vi "rtAppMain.vi"() -> ()   [LabVIEW 2012]
doc: "Top-level application."
uses:
  Typedefs/ContextID.ctl
  ContextIDFactory/ContextIDFactory.lvclass
  ContextThisComponent/ContextThisComponent.lvclass
  InvokerThisComponent/InvokerThisComponent.lvclass
  CommandFactory/CommandFactory.lvclass
  StateFactory/StateFactory.lvclass
  Model/Model/Model.lvclass
  C/Program Files (x86)/National Instruments/LabVIEW 2012/user.lib/Common/ComponentModel/ComponentModel/UserEventBasedController/UserEventBasedController.lvclass
  C/Program Files (x86)/National Instruments/LabVIEW 2012/user.lib/Common/ComponentModel/ComponentModelRT/IRQHandler/IRQHandler/IRQHandler.lvclass
  C/Program Files (x86)/National Instruments/LabVIEW 2012/user.lib/Common/ComponentModel/ComponentModelRT/RTIRQListener/RTIRQListener.lvclass
  Typedefs/CommandValue.ctl
  C/Program Files (x86)/National Instruments/LabVIEW 2012/user.lib/Common/ComponentModel/ComponentModelRT/RIOHandler/RIOHandler/RIOHandler.lvclass
  C/Program Files (x86)/National Instruments/LabVIEW 2012/user.lib/Common/ComponentModel/ComponentModelRT/LoopTimer/LoopTimer/LoopTimer.lvclass
  C/Program Files (x86)/National Instruments/LabVIEW 2012/user.lib/Common/ComponentModel/ComponentModelRT/ProgSVCmdListenerRT/ProgSVCmdListenerRT.lvclass
  Model/Target/CompactRIO/CompactRIO.lvclass
  C/Program Files (x86)/National Instruments/LabVIEW 2012/user.lib/Common/ComponentModel/ComponentModel/Heartbeat/Heartbeat/Heartbeat.lvclass
  C/Program Files (x86)/National Instruments/LabVIEW 2012/user.lib/Common/ComponentModel/ComponentModelRT/Typedefs/FPGAVIRefCRIO9074.ctl
  Typedefs/StateValue.ctl
  C/Program Files (x86)/National Instruments/LabVIEW 2012/user.lib/Common/ComponentModel/ComponentModel/Typedefs/ComponentStateValues.ctl
  Model/Model/Model.lvclass/Model.ctl
  C/Program Files (x86)/National Instruments/LabVIEW 2012/user.lib/Common/Application/AppRT9074/AppRT9074.lvclass
  Typedefs/EXATypedefs.lvlib
panel:
  out "error out":errorcluster
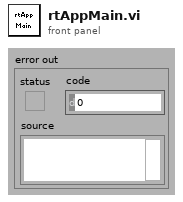
[diagram p1: front panel]
types:
  T1 = typedef "EXATypedefs.lvlib/ContextID.ctl" = enum16{"ExA"}
  T2 = typedef "EXATypedefs.lvlib/CommandValue.ctl" = enum16{"ClearError", "Disable", "Enable", "Exit", "GoToStandby", "OnHeartbeat", "OnIncomingMessagingError", "OnInterrupt", "Start"}
  T3 = typedef "componentStateValues.ctl" = enum16{"Off", "Standby", "Enabled", "Disabled", "Fault"}
  T4 = typedef "EXATypedefs.lvlib/StateValue.ctl" = enum16{"DisabledState", "EnabledState", "FaultState", "OffState", "StandbyState"}
  T5 = typedef "fpgaVIRefCRIO9074.ctl" = refnum<k20>
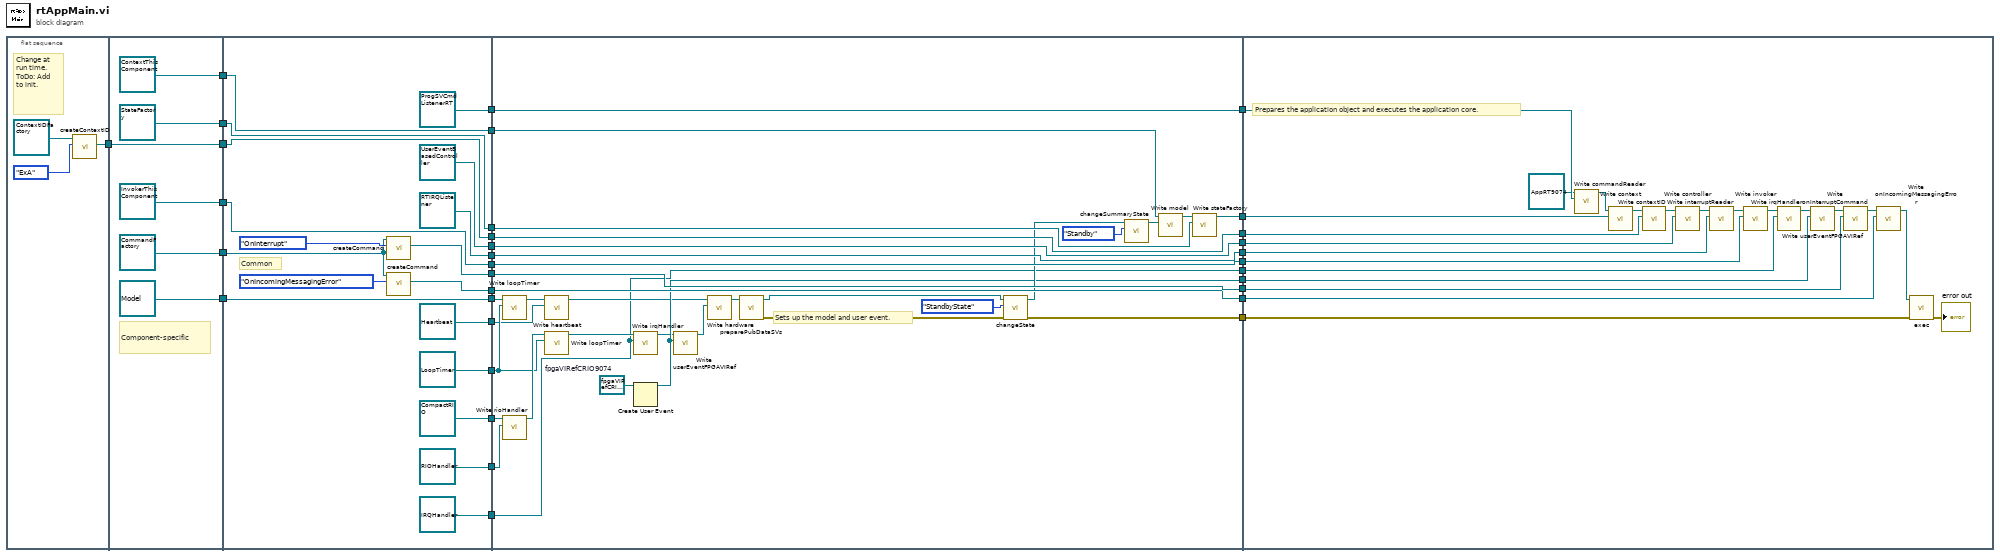
[diagram p0: block diagram]
diagram:
  n1 = flat-sequence {
    tunnel: [w35] -> w25
    tunnel: [w40] -> w28
    tunnel: [refnum<class "ContextThisComponent.lvclass"> refnum ("ConcreteContext.lvlib:ConcreteContext1.lvclass")] -> w27
    tunnel: [refnum<class "InvokerThisComponent.lvclass"> refnum ("InvokerThisComponent.lvclass")] -> w26
    tunnel: w25 -> [w40]
    tunnel: [refnum<class "CommandFactory.lvclass"> refnum ("CommandFactory.lvclass")] -> w13
    tunnel: [refnum<class "StateFactory.lvclass"> refnum ("ConcreteStateFactory.lvlib:ConcreteStateFactory.lvclass")] -> w11
    tunnel: [refnum<class "Model.lvclass"> refnum ("ConcreteModel.lvclass")] -> w9
    tunnel: [w59] -> w33
    tunnel: [w58] -> w32
    tunnel: [refnum<class "UserEventBasedController.lvclass"> refnum ("UserEventBasedController in")] -> w31
    tunnel: [refnum<class "IRQHandler.lvclass"> refnum ("IRQHandlerConcrete.lvclass")] -> w30
    tunnel: [w57] -> w29
    tunnel: w28 -> [w59]
    tunnel: w27 -> [w58]
    tunnel: w26 -> [w57]
    tunnel: [refnum<class "RTIRQListener.lvclass"> refnum ("RTIRQReader.lvclass")] -> w17
    tunnel: [refnum<class "ProgSVCmdListenerRT.lvclass"> refnum ("ProgSVCmdListenerRT.lvclass")] -> w16
    tunnel: [w55] -> w14
    tunnel: w13 -> [w45]
    tunnel: [w54] -> w12
    tunnel: w11 -> [w54]
    tunnel: [w53] -> w10
    tunnel: w9 -> [w53]
    tunnel: [refnum<class "RIOHandler.lvclass"> refnum ("RIOHandlerConcrete.lvclass")] -> w8
    tunnel: [refnum<class "LoopTimer.lvclass"> refnum ("ComponentModelRT.lvlib:LoopTimer.lvclass")] -> w7
    tunnel: [w47] -> w4
    tunnel: [refnum<class "CompactRIO.lvclass"> refnum ("CompactRIO.lvclass")] -> w2
    tunnel: [refnum<class "Heartbeat.lvclass"> refnum ("Heartbeat.lvclass")] -> w1
    tunnel: w33 -> [w93]
    tunnel: w32 -> [w83]
    tunnel: w31 -> [w91]
    tunnel: w30 -> [w61]
    tunnel: w29 -> [w92]
    tunnel: [w93] -> w24
    tunnel: [w92] -> w23
    tunnel: [w91] -> w22
    tunnel: [w74] -> w21
    tunnel: [w61] -> w20
    tunnel: [w89] -> w19
    tunnel: [w88] -> w18
    tunnel: w17 -> [w89]
    tunnel: w16 -> [w88]
    tunnel: [w87] -> w15
    tunnel: w14 -> [w87]
    tunnel: w12 -> [w85]
    tunnel: w10 -> [w71]
    tunnel: w8 -> [w72]
    tunnel: w7 -> [w67]
    tunnel: [w84] -> w6
    tunnel: [w82] -> w5
    tunnel: w4 -> [w82]
    tunnel: [w77] -> w3
    tunnel: w2 -> [w75]
    tunnel: w1 -> [w64]
    tunnel: w18 -> [w116]
    tunnel: w19 -> [w108]
    tunnel: w20 -> [w106]
    tunnel: w21 -> [w105]
    tunnel: w22 -> [w110]
    tunnel: w23 -> [w96]
    tunnel: w24 -> [w112]
    tunnel: w15 -> [w102]
    tunnel: w6 -> [w100]
    tunnel: w5 -> [w98]
    tunnel: w3 -> [w97]
    frame #0 {
      # "Change at run time.\nToDo: Add to init."
      n2 = call-dynamic "createContextID.vi"("ContextID"=ContextID."ExA", "ContextIDFactory in"=refnum<class "ContextIDFactory.lvclass"> refnum) -> ("contextID"=w35:refnum<class "ContextID.lvclass">)  [unwired: 7 in, 2 out]
    }
    frame #1 {
      # "Component-specific"
    }
    frame #2 {
      # "Common"
      n3 = call-dynamic "createCommand.vi"("commandValue"=CommandValue."OnInterrupt", "CommandFactory in"=w45) -> ("command"=w55:refnum<class "Command.lvclass">)  [unwired: 7 in, 2 out]
      n4 = call-dynamic "createCommand.vi"("commandValue"=CommandValue."OnIncomingMessagingError", "CommandFactory in"=w45) -> ("command"=w47:refnum<class "Command.lvclass">)  [unwired: 7 in, 2 out]
    }
    frame #3 {
      w90 = T5 refnum  # fpgaVIRefCRIO9074
      # "Sets up the model and user event."
      n5 = call "Write loopTimer.vi"("LoopTimer.lvclass"=w67, "Model in"=w71) -> ("Model out"=w66:refnum<class "Model.lvclass">)  [unwired: 9 in]
      n6 = call "Write rioHandler.vi"("rioHandler"=w72, "CompactRIO in"=w75) -> ("CompactRIO out"=w68:refnum<class "CompactRIO.lvclass">)  [unwired: 8 in, 1 out]
      n7 = call "Write heartbeat.vi"("IHeartbeat.lvclass"=w64, "Model in"=w66) -> ("Model out"=w65:refnum<class "Model.lvclass">)  [unwired: 9 in]
      n8 = call "Write loopTimer.vi"("ILoopTimer.lvclass"=w67, "CompactRIO in"=w68) -> ("CompactRIO out"=w63:refnum<class "CompactRIO.lvclass">)  [unwired: 9 in]
      n9 = call "Write irqHandler.vi"("irqHandler"=w61, "CompactRIO in"=w63) -> ("CompactRIO out"=w62:refnum<class "CompactRIO.lvclass">)  [unwired: 9 in]
      n10 = Create User Event(user event datatype=w90) -> (user event=w74:refnum<user-event>)  [unwired: 1 in, 1 out]
      n11 = call "Write userEventFPGAVIRef.vi"("userEventFPGAVIRef"=w74, "CompactRIO in"=w62) -> ("CompactRIO out"=w73:refnum<class "CompactRIO.lvclass">)  [unwired: 8 in, 1 out]
      n12 = call "Write hardware.vi"("Hardware.lvclass"=w73, "Model in"=w65) -> ("Model out"=w70:refnum<class "Model.lvclass">)  [unwired: 8 in, 1 out]
      n13 = call "preparePubDataSVs.vi"("Model in"=w70) -> ("error out"=w76:errorcluster, "Model out"=w80:refnum<class "Model.lvclass">)  [unwired: 9 in]
      n14 = call-dynamic "changeState.vi"("error in (no error)"=w76, "newState"=StateValue."StandbyState" ("StateValue"), "Model in"=w80) -> ("error out"=w77:errorcluster, "Model out"=w81:refnum<class "Model.lvclass">)  [unwired: 7 in]
      n15 = call-dynamic "changeSummaryState.vi"("newSummaryState"=componentStateValues."Standby" ("componentStateValues"), "Model in"=w81) -> ("Model out"=w69:refnum<class "Model.lvclass">)  [unwired: 8 in, 1 out]
      n16 = call-dynamic "Write model.vi"("Model.lvlib:Model.lvclass"=w69, "ConcreteContext1 in"=w83) -> ("ConcreteContext1 out"=w86:refnum<class "ContextThisComponent.lvclass">)  [unwired: 9 in]
      n17 = call-dynamic "Write stateFactory.vi"("StateFactory.lvlib:StateFactory.lvclass"=w85, "ConcreteContext1 in"=w86) -> ("ConcreteContext1 out"=w84:refnum<class "ContextThisComponent.lvclass">)  [unwired: 9 in]
    }
    frame #4 {
      # "Prepares the application object and executes the application core."
      n18 = call "Write commandReader.vi"("commandReader"=w116, "AppRT9074 in"=refnum<class "AppRT9074.lvclass"> refnum) -> ("AppRT9074 out"=w114:refnum<class "AppRT9074.lvclass">)  [unwired: 8 in, 1 out]
      n19 = call "Write context.vi"("context"=w100, "AppRT9074 in"=w114) -> ("AppRT9074 out"=w113:refnum<class "AppRT9074.lvclass">)  [unwired: 8 in, 1 out]
      n20 = call "Write contextID.vi"("contextID"=w112, "AppRT9074 in"=w113) -> ("AppRT9074 out"=w111:refnum<class "AppRT9074.lvclass">)  [unwired: 8 in, 1 out]
      n21 = call "Write controller.vi"("controller"=w110, "AppRT9074 in"=w111) -> ("AppRT9074 out"=w109:refnum<class "AppRT9074.lvclass">)  [unwired: 8 in, 1 out]
      n22 = call "Write interruptReader.vi"("interruptReader"=w108, "AppRT9074 in"=w109) -> ("AppRT9074 out"=w95:refnum<class "AppRT9074.lvclass">)  [unwired: 8 in, 1 out]
      n23 = call "Write invoker.vi"("invoker"=w96, "AppRT9074 in"=w95) -> ("AppRT9074 out"=w107:refnum<class "AppRT9074.lvclass">)  [unwired: 8 in, 1 out]
      n24 = call "Write irqHandler.vi"("irqHandler"=w106, "AppRT9074 in"=w107) -> ("AppRT9074 out"=w101:refnum<class "AppRT9074.lvclass">)  [unwired: 8 in, 1 out]
      n25 = call "Write userEventFPGAVIRef.vi"("userEventFPGAVIRef"=w105, "AppRT9074 in"=w101) -> ("AppRT9074 out"=w103:refnum<class "AppRT9074.lvclass">)  [unwired: 8 in, 1 out]
      n26 = call "Write onInterruptCommand.vi"("onInterruptCommand"=w102, "AppRT9074 in"=w103) -> ("AppRT9074 out"=w94:refnum<class "AppRT9074.lvclass">)  [unwired: 8 in, 1 out]
      n27 = call "Write onIncomingMessagingError.vi"("Command.lvclass"=w98, "AppRT9074 in"=w94) -> ("AppRT9074 out"=w99:refnum<class "AppRT9074.lvclass">)  [unwired: 8 in, 1 out]
      n28 = call-dynamic "exec.vi"("error in (no error)"=w97, "AppRT9074 in"=w99) -> ("error out"=→"error out":errorcluster)  [unwired: 8 in, 1 out]
    }
  }
